vi "Assert NoError.vi"(9 "error in (no error)":errorcluster, 10 "Assert Number":T1 items=["LabVIEW Internal Error"]) -> (1 "error out":errorcluster)   [LabVIEW 2017, in "WebServiceImporter.lvlib" / "Error Handling.lvlib"]
uses:
  <vilib>/Platform/WebService/Error Handling/Error Handling.lvlib
  <vilib>/Platform/WebService/Error Handling/Assert/Assert Number.ctl
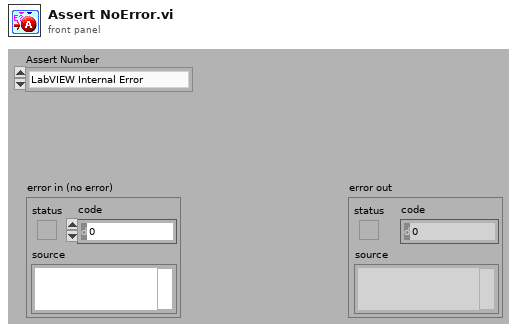
[diagram p1: front panel]
types:
  T1 = typedef "WebServiceImporter.lvlib/Error Handling.lvlib/Assert Number.ctl" = u16
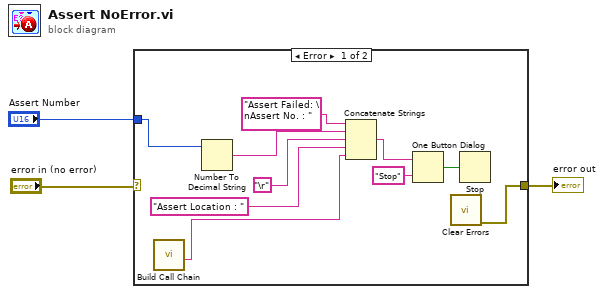
[diagram p0: block diagram]
diagram:
  n1 = case shown="Error" "error in (no error)" {
    selector: "error in (no error)" -> [_ w14]
    tunnel: "Assert Number" -> [w5 _]
    tunnel: [w4 w14] -> w1
    frame Error {
      n2 = call <vilib>:"Build Call Chain.vi"() -> ("Call Chain"=w12:string)  [unwired: 11 in]
      n3 = Number To Decimal String(number=w5) -> (decimal integer string=w9:string)  [unwired: 1 in]
      n4 = Concatenate Strings("Assert Failed: \nAssert No. : ", w9, "\r", "Assert Location : ", w12) -> (w13:string)
      n5 = One Button Dialog(message=w13, button name ("OK")="Stop") -> (true=w7:bool)
      n6 = call <vilib>:"Clear Errors.vi"() -> ("error out"=w4:errorcluster)  [unwired: 6 in, 1 out]
      n7 = Stop(stop? (T)=w7) -> ()
    }
    frame No Error {
    }
  }
  "error out" <- w1
